vi "GlobalActuators.vi"() -> ()   [LabVIEW 2020]
panel:
  out "REF_Motor1":string
  # "DEVICE REFERENCE NAMES"
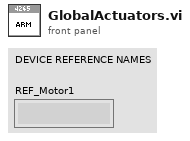
[diagram p1: front panel]
diagram:
